vi "3D Cartesian Coordinate Rotation (Direction).vi"   [LabVIEW 2012, in "NI_AALPro.lvlib"]
doc: "Rotates a three-dimensional Cartesian coordinate in the counterclockwise direction using the direction cosines method. Wire data to the <B>X</B> input to determine the polymorphic instance to use or manually select the instance."
uses:
  NI_AALPro.lvlib
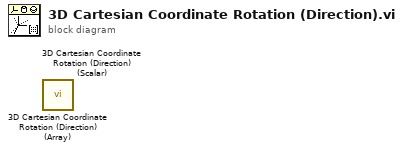
[diagram p0: block diagram]
diagram:
  n1 = call "3D Cartesian Coordinate Rotation (Direction) (Array).vi"() -> ()  [unwired: 8 in, 4 out]
  n2 = call "3D Cartesian Coordinate Rotation (Direction) (Scalar).vi"() -> ()  [unwired: 8 in, 4 out]
